vi "Read Right.vi"(2 "error in (no error)":errorcluster, 3 "Rectangle.lvclass":refnum<class "Rectangle.lvclass">) -> (0 "error out":errorcluster, 1 "Bottom":dbl)   [LabVIEW 2015, in "Rectangle.lvclass"]
uses:
  Rectangle.lvclass
  Rectangle.lvclass/Rectangle.ctl
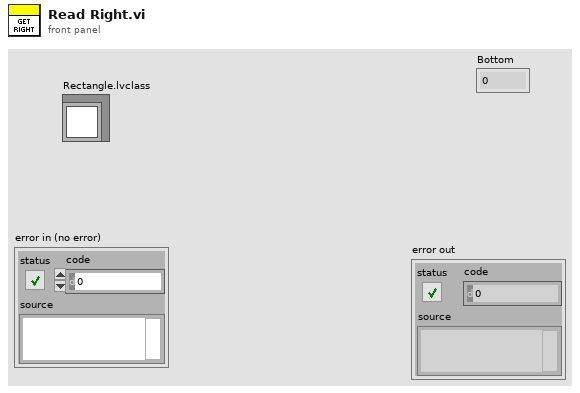
[diagram p1: front panel]
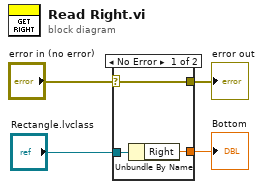
[diagram p0: block diagram]
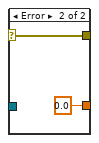
[diagram p2: hidden frame]
diagram:
  n1 = case shown="No Error" "error in (no error)" {
    selector: "error in (no error)" -> [w7 w9]
    tunnel: [w7 w9] -> w3
    tunnel: "Rectangle.lvclass" -> [w6 _]
    tunnel: [w5 0.0] -> w1
    frame No Error {
      n2 = Unbundle By Name(w6) -> ("Right"=w5:dbl)
    }
    frame Error {
    }
  }
  "error out" <- w3
  "Bottom" <- w1
